vi "Test Get Latest Message Contet Correct.vi"(8 "error in (no error)":errorcluster, 11 "Test Case In":refnum<class "Debugger Test.lvclass">) -> (0 "error out":errorcluster, 3 "Test Case Out":refnum<class "Debugger Test.lvclass">)   [LabVIEW 2020, in "Debugger Test.lvclass"]
uses:
  Debugger Test.lvclass
  C:/Program Files (x86)/National Instruments/LabVIEW 2020/vi.lib/Astemes/LUnit/Test Case.lvclass
  source/Debugger/Debugger.lvclass
  C:/Users/anton/Documents/GitHub/triarc-debugger/source/Process/Debug Process.lvclass
  source/Debug Data/Raw Debug Data.ctl
  source/Process/Debug Process.lvclass/Debug Process.ctl
  source/Debug Data/Debug Data.lvclass/Debug Data.ctl
  <vilib>/Astemes/LUnit/Test Case.lvclass/Test Case.ctl
  <vilib>/Astemes/LUnit/LUnit Assertion Result.lvclass/LUnit Assertion Result.ctl
  <vilib>/Astemes/LUnit/LUnit Test Case Result.lvclass/LUnit Test Case Result.ctl
  <vilib>/Astemes/LUnit/LUnit Method Result.lvclass/LUnit Method Result.ctl
  01074fa8-ee8a-411d-bc8b-fc92c4f90959.vi
  source/Process/Public/Lifecycle/Get Lifecycle State.vi
  <vilib>/AdvancedString/Delimited String to 1D String Array.vi
  <vilib>/Astemes/Triarc Framework/Broadcast Event Helpers/Execution timer.vi
  source/Process/Private/SubVIs/Wait for finish.vi
  source/Process/Protected/Messaging/Enqueue Message.vi
  source/Process/Private/SubVIs/Set Lifecycle State.vi
  <vilib>/Astemes/LUnit/Palette/Pass.vi
  <vilib>/Astemes/LUnit/Palette/Fail.vi
  <vilib>/Astemes/LUnit/Compare Variants.vi
  <vilib>/Astemes/LUnit/Describe Comparison.vi
  <vilib>/Astemes/LUnit/Set Assertion Type.vi
  <vilib>/Utility/error.llb/Clear Errors.vi
  <vilib>/Astemes/LUnit/Add test result.vi
  <vilib>/Astemes/LUnit/LUnit Write Passed.vi
  <vilib>/Astemes/LUnit/LUnit Write Message.vi
  <vilib>/Astemes/LUnit/LUnit Write Description.vi
  <vilib>/Astemes/LUnit/Variant to string.vi
  <vilib>/Astemes/LUnit/LUnit Write Assertion Type.vi
  <vilib>/Astemes/LUnit/LUnit Record Assertion Result.vi
  <vilib>/Astemes/LUnit/LUnit Aggregate Assertion Results.vi
  <vilib>/Astemes/LUnit/Assertion Result/LUnit Read Status.vi
  <vilib>/Astemes/LUnit/LUnit Read Message.vi
  <vilib>/Astemes/LUnit/LUnit Read Description.vi
  <vilib>/Astemes/LUnit/Method Result/LUnit Merge Status.vi
  <vilib>/Astemes/LUnit/LUnit Concatenate result strings.vi
  <vilib>/Utility/error.llb/Error Cluster From Error Code.vi
  <vilib>/Astemes/Triarc Framework/Broadcast Event Helpers/Dequeue Broadcast Message.vi
  <vilib>/Utility/Data Type/Get Type Information.vi
  <vilib>/Utility/LVClass/Get LV Class Name.vi
  source/Debug Data/Debug Data.lvclass
  <vilib>/Astemes/LUnit/LUnit Assertion Result.lvclass
  source/Process/Debug Process.lvclass
  <vilib>/Astemes/Triarc Framework/Broadcast Event Helpers/Broadcast Event Helpers.lvlib
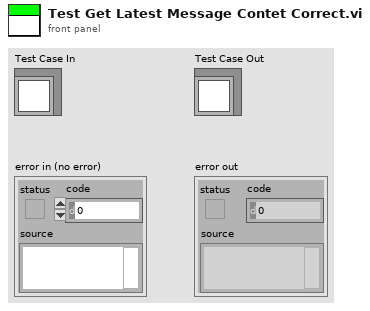
[diagram p1: front panel]
types:
  T1 = typedef "Debug Data.lvclass/Raw Debug Data.ctl" = cluster{"Action":string, "Call Chain":string, "Process":string, "Message":string, "Message Data":variant, "Time":dbl}
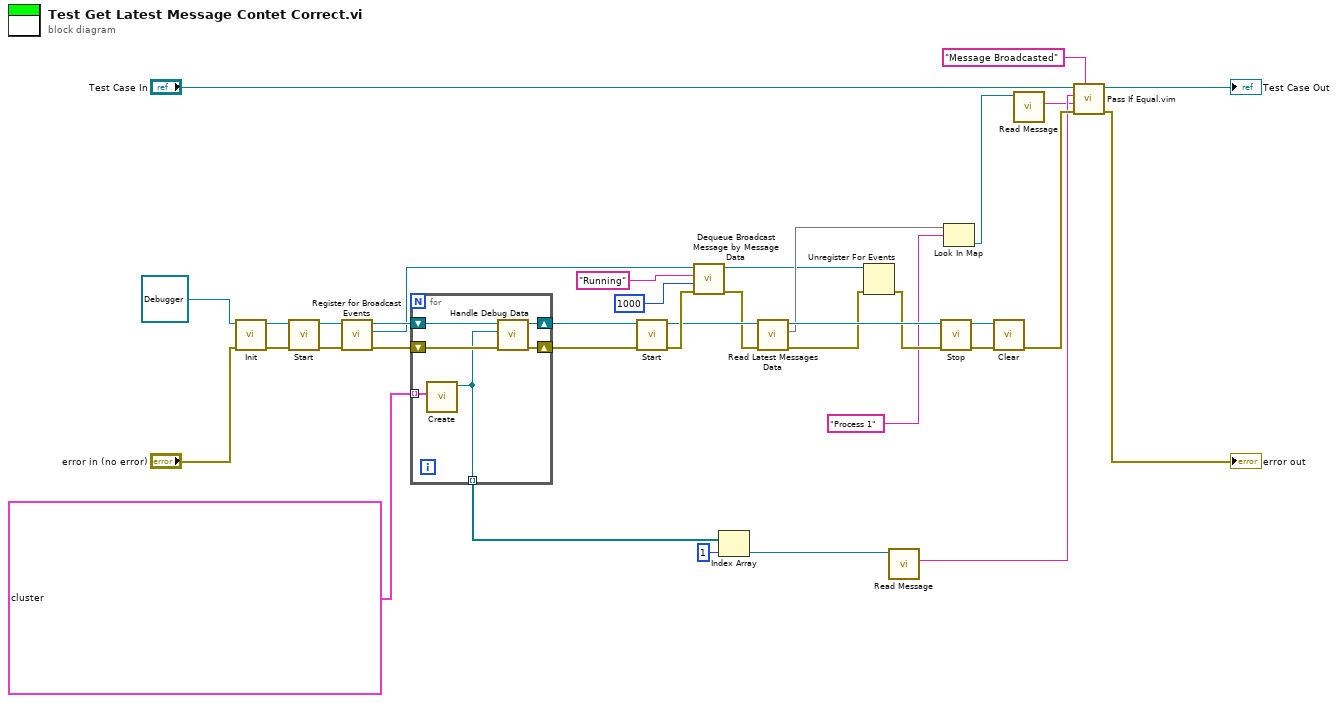
[diagram p0: block diagram]
diagram:
  n1 = call-dynamic "Init.vi"("error in (no error)"="error in (no error)", "Process In"=refnum<class "Debugger.lvclass"> refnum ("Debug Data Event In 2")) -> ("error out"=w32:errorcluster, "Process Out"=w33:refnum<class "Debugger.lvclass">)  [unwired: 8 in]
  n2 = call "Start.vi"("error in (no error)"=w32, "Process In"=w33) -> ("error out"=w30:errorcluster, "Process Out"=w31:refnum<class "Debugger.lvclass">)  [unwired: 7 in, 1 out]
  n3 = call "Register for Broadcast Events.vi"("error in (no error)"=w30, "Process In"=w31) -> ("error out"=w29:errorcluster, "Event Registration Refnum Out"=w4:refnum<event-registration>, "Process Out"=w24:refnum<class "Debugger.lvclass">)  [unwired: 7 in]
  n4 = for {
    shift-right: [w40] -> w28
    shift-left: w29 -> [w42]
    shift-right: [w41] -> w10
    shift-left: w24 -> [w39]
    tunnel: T1[] [{"Action"="Send", "Call Chain"="Test.vi:123456", "Process"="Process 1", "Message"="Init", "Message Data"=variant, "Time"=0.0}, {"Action"="Receive", "Call Chain"="TF.lvlib:Process.lvclass:Handle Messages.vi:1960001", "Process"="Process 1", "Message"="Init", "Message Data"=variant, "Time"=0.0}, {"Action"="Send", "Call Chain"="Test.vi", "Process"="Process 1", "Message"="Start", "Message Data"=variant, "Time"=0.0}] ("Debug Data Cluster") -> [w38] mode=indexing
    tunnel: [w37] -> w12 mode=indexing
    n5 = call "Create.vi"("Debug Data Cluster"=w38) -> ("Debug Data out"=w37:refnum<class "Debug Data.lvclass">)  [unwired: 9 in, 1 out]
    n6 = call-dynamic "Handle Debug Data.vi"("error in (no error)"=w42, "Debug Data.lvclass"=w37, "Debug Data Event In"=w39) -> ("error out"=w40:errorcluster, "Debug Data Event Out"=w41:refnum<class "Debugger.lvclass">)  [unwired: 7 in]
  }
  n7 = call "Start.vi"("error in (no error)"=w28, "Process In"=w10) -> ("error out"=w11:errorcluster, "Process Out"=w9:refnum<class "Debugger.lvclass">)  [unwired: 7 in, 1 out]
  n8 = call <vilib>:"Dequeue Broadcast Message by Message Data.vi"("error in (no error)"=w11, "Timeout (-1)"=1000, "Message Data"="Running", "Event Registration Refnum"=w4) -> ("error out"=w5:errorcluster, "Event Registration Refnum Out"=w3:refnum<event-registration>)  [unwired: 3 in, 3 out]
  n9 = Index Array(array=w12, index=1) -> (element=w16:refnum<class "Debug Data.lvclass">)
  n10 = call "Read Latest Messages Data.vi"("error in (no error)"=w5, "Debugger In"=w9) -> ("error out"=w19:errorcluster, "Latest Messages"=w8:map{string, refnum<class "Debug Data.lvclass">}, "Debugger Out"=w27:refnum<class "Debugger.lvclass">)  [unwired: 7 in]
  n11 = Unregister For Events(event registration refnum=w3, error in=w19) -> (error out=w18:errorcluster)
  n12 = call "Read Message.vi"("Debug Data in"=w16) -> ("Message"=w7:string)  [unwired: 8 in, 2 out]
  n13 = call "Stop.vi"("error in (no error)"=w18, "Process In"=w27) -> ("error out"=w25:errorcluster, "Process Out"=w26:refnum<class "Debugger.lvclass">)  [unwired: 7 in, 1 out]
  n14 = Look In Map(map=w8, key="Process 1") -> (value=w15:refnum<class "Debug Data.lvclass">)  [unwired: 1 in, 1 out]
  n15 = call-dynamic "Clear.vi"("error in (no error)"=w25, "Process In"=w26) -> ("error out"=w21:errorcluster)  [unwired: 9 in]
  n16 = call "Read Message.vi"("Debug Data in"=w15) -> ("Message"=w6:string)  [unwired: 8 in, 2 out]
  n17 = call "Pass If Equal.vim"("Description"="Message Broadcasted", "error in (no error)"=w21, "Actual"=w6, "Expected"=w7, "LUnit Test Case In"="Test Case In") -> ("error out"=→"error out":errorcluster, "LUnit Test Case Out"=→"Test Case Out":refnum<class "Debugger Test.lvclass">)  [unwired: 5 in]
